vi "CreatePathWriteTrajCSVFile_Example.vi"(11 "Max Velocity M/S":dbl=3.2 format="%17.3f") -> (1 "PathPlannerTrajectory":T2 {"States"."TargetHolonomicRotation"."SIN" format="%13.4f"; "States"."TargetHolonomicRotation"."COS" format="%13.4f"; "States"."TargetHolonomicRotation"."VALUE" format="%13.4f"; "States"."Heading"."SIN" format="%13.4f"; "States"."Heading"."COS" format="%13.4f"; "States"."Heading"."VALUE" format="%13.4f"; "States"."PositionMeters"."Y" format="%14.3f"; "States"."PositionMeters"."X" format="%14.3f"}, 2 "Trajectory State\nCount":i32, 3 "TotalTImeSecs":dbl)   [LabVIEW 2019]
uses:
  <vilib>/Rock Robotics/WPI/ThirdParty/MJansen/PathPlanner/TypeDef/PathPlannerTrajectory.ctl
  <vilib>/Rock Robotics/WPI/ThirdParty/MJansen/PathPlanner/TypeDef/PathPlannerTrajectoryState.ctl
  <vilib>/Rock Robotics/WPI/ThirdParty/JAS_Junk/TrajLib/TypeDef/TRANSLATION2D.ctl
  <vilib>/Rock Robotics/WPI/ThirdParty/JAS_Junk/TrajLib/TypeDef/ROTATION2D.ctl
  <vilib>/Rock Robotics/WPI/ThirdParty/MJansen/PathPlanner/TypeDef/PathPlannerPathConstraints.ctl
  <vilib>/Rock Robotics/WPI/ThirdParty/JAS_Junk/TrajLib/Rotation2d_CreateAngle.vi
  <vilib>/Rock Robotics/WPI/ThirdParty/JAS_Junk/TrajLib/Translation2d_Create.vi
  <vilib>/Rock Robotics/WPI/ThirdParty/JAS_Junk/TrajLib/Pose2d_getTranslation.vi
  <vilib>/Rock Robotics/WPI/ThirdParty/JAS_Junk/TrajLib/Translation2d_GetDistance.vi
  <vilib>/Rock Robotics/WPI/ThirdParty/JAS_Junk/TrajLib/Pose2d_getRotation.vi
  <vilib>/Rock Robotics/WPI/ThirdParty/JAS_Junk/TrajLib/Translation2d_Create_DistAng.vi
  <vilib>/Rock Robotics/WPI/ThirdParty/JAS_Junk/TrajLib/Translation2d_Plus.vi
  <vilib>/Rock Robotics/WPI/ThirdParty/JAS_Junk/TrajLib/Rotation2d_Plus.vi
  <vilib>/Rock Robotics/WPI/ThirdParty/JAS_Junk/TrajLib/Util_CalcDist.vi
  <vilib>/Rock Robotics/WPI/ThirdParty/JAS_Junk/TrajLib/Rotation2d_GetAngleCosSin.vi
  <vilib>/Rock Robotics/WPI/ThirdParty/JAS_Junk/TrajLib/Rotation2d_RotateBy.vi
  <vilib>/Rock Robotics/WPI/ThirdParty/JAS_Junk/TrajLib/Rotation2d_CreateXY.vi
  <vilib>/Rock Robotics/WPI/ThirdParty/MJansen/PathPlanner/PathPlanner24.lvlib
  <vilib>/Rock Robotics/WPI/ThirdParty/JAS_Junk/TrajLib/Trajectory_Library.lvlib
panel:
  in  "Trajectory CSV File Name":path=path "sample.csv"
  in  "Optional Comment":string="Sample PathPlanner Trajectory"
  in  "Write File":bool
  out "Trajectory\nWrite error":errorcluster
  in  "End Angle Degrees":dbl format="%#_13g"
  in  "End Velocity M/S":dbl format="%#_13g"
  in  "Start Angual Vel Rad/S":dbl format="%#_13g"
  in  "Start Y Vel M/S":dbl format="%#_13g"
  in  "Start X Vel M/S":dbl format="%#_13g"
  in  "MaxAngularAccel Radians.Sec^2":dbl=2.4 format="%17.3f"
  in  "Point 4":T1={"X Meters"=3.0, "Y Meters"=3.0, "Heading  Deg"=90.0} {"Heading  Deg" format="%13.3f"; "Y Meters" format="%13.3f"; "X Meters" format="%13.3f"}
  in  "Point 3":T1={"X Meters"=3.0, "Y Meters"=2.7, "Heading  Deg"=90.0} {"Heading  Deg" format="%13.3f"; "Y Meters" format="%13.3f"; "X Meters" format="%13.3f"}
  in  "Point 2":T1={"X Meters"=1.3, "Y Meters"=1.0, "Heading  Deg"=0.0} {"Heading  Deg" format="%13.3f"; "Y Meters" format="%13.3f"; "X Meters" format="%13.3f"}
  out "Path\nCreation\nError":bool
  out "Trajectory":cluster{dbl[], dbl[]}(graph)
  in  "Initial Point":T1={"X Meters"=1.0, "Y Meters"=1.0, "Heading  Deg"=0.0} {"Heading  Deg" format="%13.3f"; "Y Meters" format="%13.3f"; "X Meters" format="%13.3f"}
  in  "MaxAcceleration M/S^2":dbl=2.8 format="%17.1f"
  in  "MaxAngularVel  Radians/Sec":dbl=1.8 format="%17.3f"
  # "Create PathPlanner Path/Trajectory Sample"
  # "This VI is designed to be called by BEGIN.VI, but can be executed directly to test trajectory parameters."
  # "CREATED TRAJECTORY INFORMATION"
  # "PATH CONFIGURATION"
  # "PATH DEFINITION"
  # "WRITE TRAJECTORY TO FILE"
  # "There can be as many points as needed."
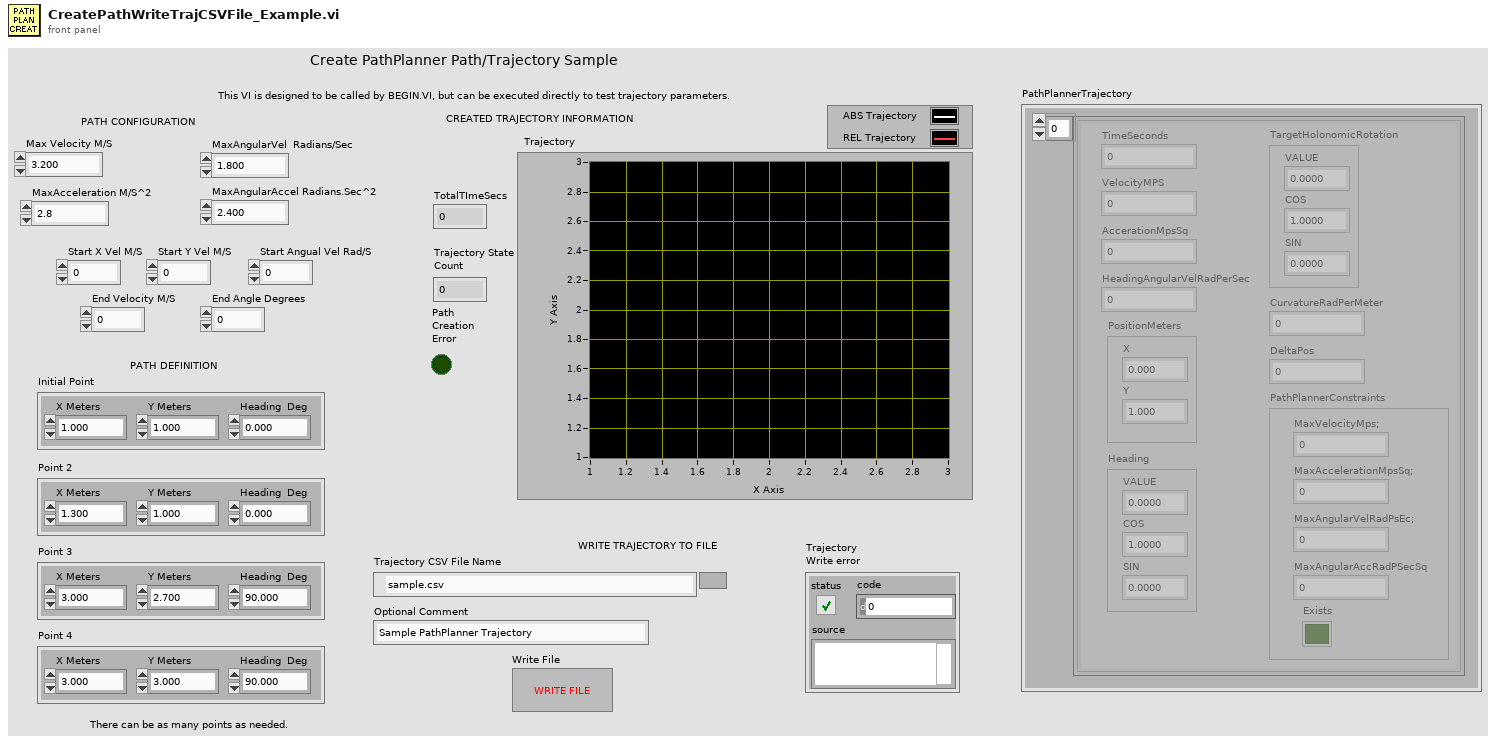
[diagram p1: front panel]
types:
  T1 = cluster{"X Meters":dbl, "Y Meters":dbl, "Heading  Deg":dbl}
  T2 = typedef "PathPlanner24.lvlib/PathPlannerTrajectory.ctl" = cluster{"States":T3[]}
  T3 = typedef "PathPlanner24.lvlib/PathPlannerTrajectoryState.ctl" = cluster{"TimeSeconds":dbl, "VelocityMPS":dbl, "AccerationMpsSq":dbl, "HeadingAngularVelRadPerSec":dbl, "PositionMeters":T4, "Heading":T5, "TargetHolonomicRotation":T5, "CurvatureRadPerMeter":dbl, "PathPlannerConstraints":T6, "DeltaPos":dbl}
  T4 = typedef "Trajectory_Library.lvlib/TRANSLATION2D.ctl" = cluster{"X":dbl, "Y":dbl}
  T5 = typedef "Trajectory_Library.lvlib/ROTATION2D.ctl" = cluster{"VALUE":dbl, "COS":dbl, "SIN":dbl}
  T6 = typedef "PathPlanner24.lvlib/PathPlannerPathConstraints.ctl" = cluster{"MaxVelocityMps;":dbl, "MaxAccelerationMpsSq;":dbl, "MaxAngularVelRadPsEc;":dbl, "MaxAngularAccRadPSecSq":dbl, "Exists":bool}
  T7 = typedef "Trajectory_Library.lvlib/POSE2D.ctl" = cluster{"TRANSLATION":T4, "ROTATION":T5}
  T8 = typedef "Trajectory_Library.lvlib/CHASSIS_SPEEDS.ctl" = cluster{"vX":dbl, "vY":dbl, "vOmega":dbl}
  T9 = typedef "PathPlanner24.lvlib/PathPlannerGoalEndState.ctl" = cluster{"Velocity":dbl, "Rotation":T5}
  T10 = typedef "PathPlanner24.lvlib/PathPlannerPath.ctl" = cluster{"BezierPoints":T4[], "PreviewStartingRotation":T5, "Reversed":bool, "RotationTargets":T11[], "ConstraintZones":T12[], "EventMarkers":T13[], "GlobalConstraints":T6, "GoalEndState":T9, "AllPoints":T16[]}
  T11 = typedef "PathPlanner24.lvlib/PathPlannerRotationTarget.ctl" = cluster{"target":T5, "WaypointRelativePosition":dbl, "Exists":bool}
  T12 = typedef "PathPlanner24.lvlib/PathPlannerConstraintsZone.ctl" = cluster{"minWaypointPos":dbl, "maxWaypointPos":dbl, "Constraints":T6, "Present":bool}
  T13 = typedef "PathPlanner24.lvlib/PathPlannerEventMarker.ctl" = cluster{"WaypointRelativePos":dbl, "minimumTriggerDistance":dbl, "markerPos":T4, "lastRobotPos":T4, "Command":T14, "markerPos Exists":bool, "LastRobotPoseExists":bool}
  T14 = typedef "PathPlanner24.lvlib/PathPlannerCommandUtil.ctl" = cluster{"waitTime":dbl, "name":string, "pathName":string, "commands":cluster{"type":string, "waitTime":dbl, "name":string, "pathName":string}[], "type":T15}
  T15 = typedef "PathPlanner24.lvlib/PathPlanner_CommandUtilType_ENUM.ctl" = enum16{"Unknown", "Wait", "Named", "Path", "Sequential", "Parallel", "Race", "Deadline"}
  T16 = typedef "PathPlanner24.lvlib/PathPlannerPathPoint.ctl" = cluster{"Position":T4, "HolonomicRotation":T5, "DistAlongPath":dbl, "CurveRadius":dbl, "MaxV":dbl, "Constraints":T6, "HolonomicRotationExists":bool}
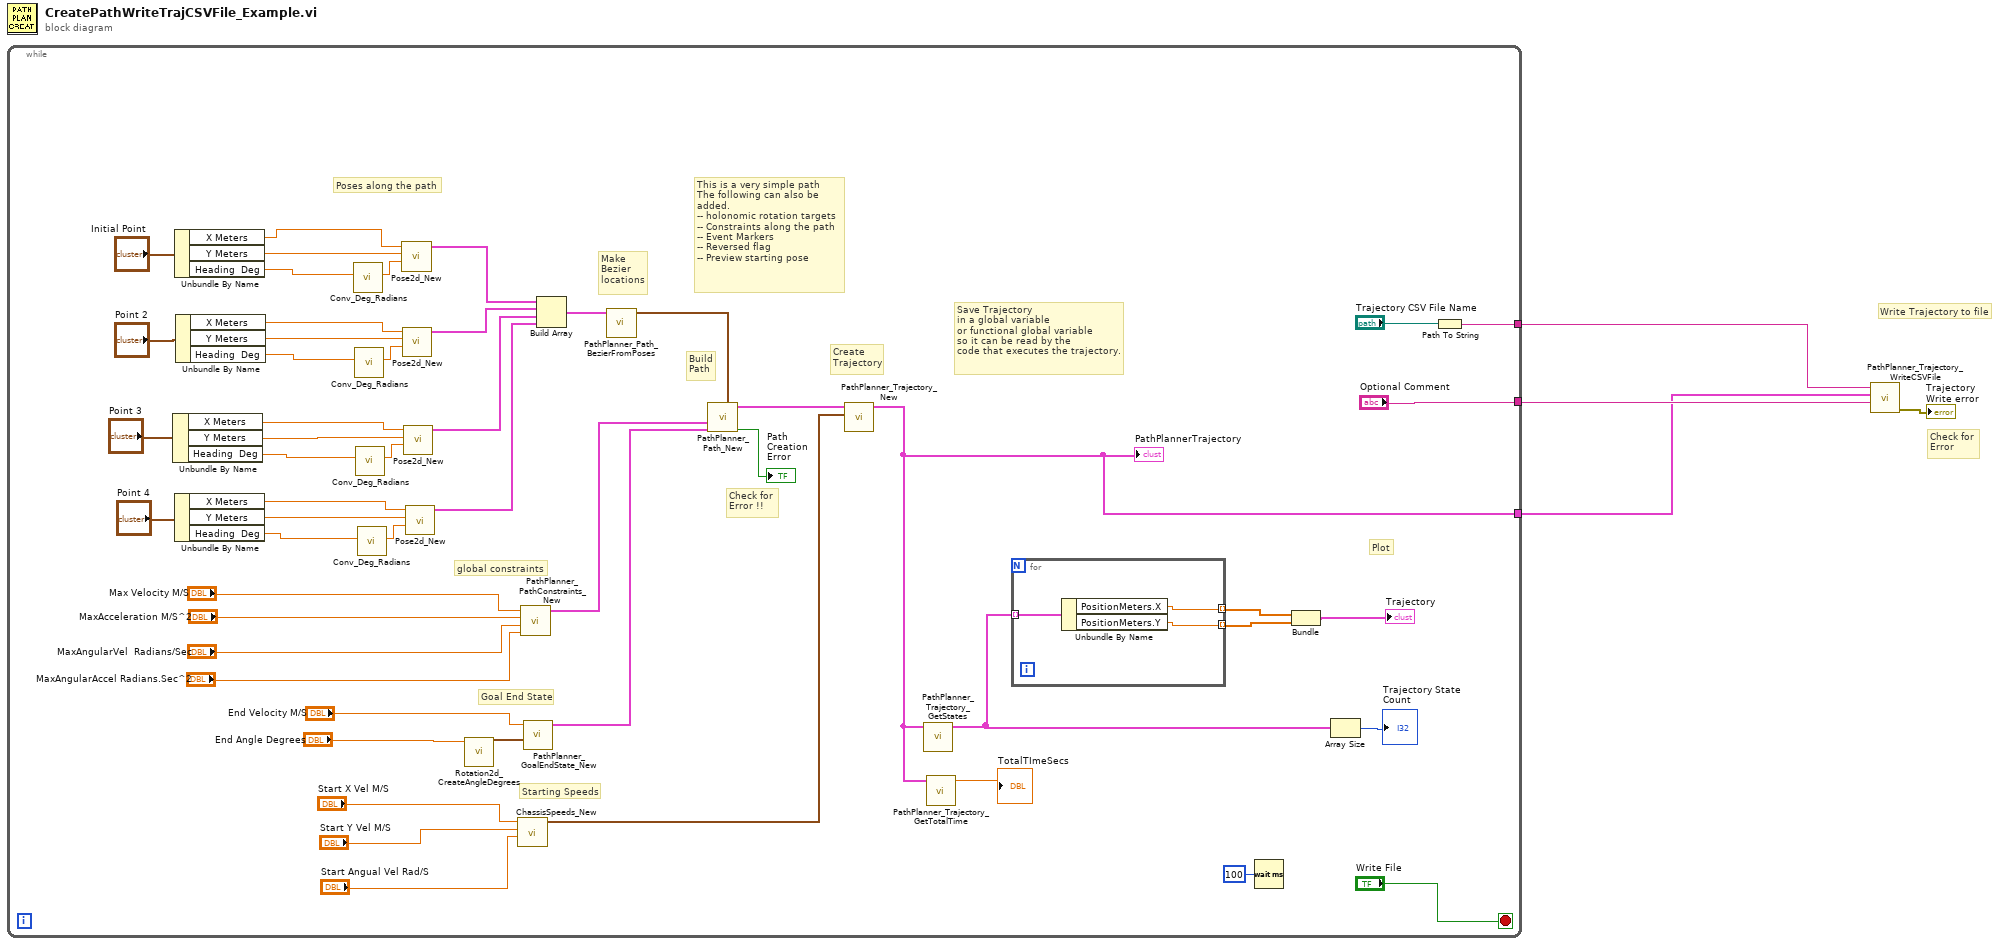
[diagram p0: block diagram]
diagram:
  # "Write Trajectory to file"
  # "Check for\nError"
  n1 = while {
    tunnel: ["Optional Comment"] -> w3
    tunnel: [w7] -> w2
    tunnel: [w6] -> w1
    stop <- "Write File" stop-if-true
    # "This is a very simple path\nThe following can also be\nadded.\n-- holonomic rotation targets\n-- Constraints along the path\n-- Event Markers\n-- Reversed flag\n-- Preview starting pose"
    # "Plot"
    # "Save Trajectory\nin a global variable\nor functional global variable\nso it can be read by the \ncode that executes the trajectory."
    # "Create\nTrajectory"
    # "Check for\nError !!"
    # "Starting Speeds"
    # "Goal End State"
    # "global constraints"
    # "Make\nBezier\nlocations"
    # "Build\nPath"
    # "Poses along the path"
    n2 = Unbundle By Name("Point 3") -> ("X Meters"=w20:dbl, "Y Meters"=w19:dbl, "Heading  Deg"=w18:dbl)
    n3 = Unbundle By Name("Initial Point") -> ("X Meters"=w28:dbl, "Y Meters"=w27:dbl, "Heading  Deg"=w26:dbl)
    n4 = Unbundle By Name("Point 4") -> ("X Meters"=w17:dbl, "Y Meters"=w16:dbl, "Heading  Deg"=w15:dbl)
    n5 = Unbundle By Name("Point 2") -> ("X Meters"=w25:dbl, "Y Meters"=w24:dbl, "Heading  Deg"=w23:dbl)
    n6 = call <vilib>:"Conv_Deg_Radians.vi"("Degress"=w26) -> ("Radians"=w37:dbl)  [unwired: 10 in]
    n7 = call <vilib>:"Conv_Deg_Radians.vi"("Degress"=w23) -> ("Radians"=w38:dbl)  [unwired: 10 in]
    n8 = call <vilib>:"Conv_Deg_Radians.vi"("Degress"=w18) -> ("Radians"=w39:dbl)  [unwired: 10 in]
    n9 = call <vilib>:"Conv_Deg_Radians.vi"("Degress"=w15) -> ("Radians"=w40:dbl)  [unwired: 10 in]
    n10 = call <vilib>:"Pose2d_New.vi"("Heading"=w37, "Y"=w27, "X"=w28) -> ("out POSe"=w41:T7)  [unwired: 8 in]
    n11 = call <vilib>:"Pose2d_New.vi"("Heading"=w38, "Y"=w24, "X"=w25) -> ("out POSe"=w42:T7)  [unwired: 8 in]
    n12 = call <vilib>:"Pose2d_New.vi"("Heading"=w39, "Y"=w19, "X"=w20) -> ("out POSe"=w43:T7)  [unwired: 8 in]
    n13 = call <vilib>:"Pose2d_New.vi"("Heading"=w40, "Y"=w16, "X"=w17) -> ("out POSe"=w44:T7)  [unwired: 8 in]
    n14 = call <vilib>:"Rotation2d_CreateAngleDegrees.vi"("Angle_Degrees"="End Angle Degrees") -> ("ROTATION"=w48:T5)  [unwired: 10 in]
    n15 = call <vilib>:"ChassisSpeeds_New.vi"("vAngular"="Start Angual Vel Rad/S", "vY"="Start Y Vel M/S", "vX"="Start X Vel M/S") -> ("CHASSIS"=w56:T8)  [unwired: 8 in]
    n16 = call <vilib>:"PathPlanner_PathConstraints_New.vi"("MaxAngularAccRadPSecSq"="MaxAngularAccel Radians.Sec^2", "MaxAngularVelRadPsEc;"="MaxAngularVel  Radians/Sec", "MaxAccelerationMpsSq;"="MaxAcceleration M/S^2", "MaxVelocityMps;"="Max Velocity M/S") -> ("PathPlannerConstraints"=w46:T6)  [unwired: 7 in]
    n17 = call <vilib>:"PathPlanner_GoalEndState_New.vi"("Rotation"=w48, "Velocity"="End Velocity M/S") -> ("GoalEndState"=w50:T9)  [unwired: 9 in]
    n18 = Build Array(w41, w42, w43, w44) -> (w36:T7[])
    n19 = call <vilib>:"PathPlanner_Path_BezierFromPoses.vi"("Poses"=w36) -> ("Bezier"=w45:T4[])  [unwired: 9 in, 1 out]
    n20 = call <vilib>:"PathPlanner_Path_New.vi"("BezierPoints"=w45, "GoalEndState"=w50, "GlobalConstraints"=w46) -> ("Error"=→"Path\nCreation\nError":bool, "PathPlannerPath"=w52:T10)  [unwired: 7 in]
    n21 = call <vilib>:"PathPlanner_Trajectory_New.vi"("StartingSpeeds"=w56, "Path"=w52) -> ("PathPlannerTrajectory"=w6:T2)  [unwired: 9 in]
    "PathPlannerTrajectory" <- w6
    n22 = call <vilib>:"PathPlanner_Trajectory_GetStates.vi"("PathPlannerTrajectory"=w6) -> ("PathPlannerStates"=w32:T3[])  [unwired: 10 in]
    n23 = call <vilib>:"PathPlanner_Trajectory_GetTotalTime.vi"("PathPlannerTrajectory"=w6) -> ("TotalTimeSeconds"=→"TotalTImeSecs":dbl)  [unwired: 10 in]
    n24 = for {
      tunnel: [w60] -> w34 mode=indexing
      tunnel: [w59] -> w35 mode=indexing
      tunnel: w32 -> [w58] mode=indexing
      n25 = Unbundle By Name(w58) -> ("PositionMeters.X"=w60:dbl, "PositionMeters.Y"=w59:dbl)
    }
    n26 = Wait (ms)(milliseconds to wait=u32 100) -> ()  [unwired: 1 out]
    n27 = Bundle(w34, w35) -> (→"Trajectory":cluster{dbl[], dbl[]})  [unwired: 1 in]
    n28 = Array Size(array=w32) -> (size(s)=→"Trajectory State\nCount":i32)
    n29 = Path To String(path="Trajectory CSV File Name") -> (string=w7:string)
  }
  n30 = call <vilib>:"PathPlanner_Trajectory_WriteCSVFile.vi"("Comment"=w3, "TRAJECTORY"=w1, "FileName"=w2) -> ("error out"=→"Trajectory\nWrite error":errorcluster)  [unwired: 8 in]
